vi "Create Core.vi"(6 "Custom Config Data":u8[](array[numeric]) format="%.0x", 7 "Direction":T2, 8 "error in (no error)":errorcluster, 9 "Disconnect Behavior":T1, 10 "Name":string, 11 "CIFChannels in":refnum<class "CIFChannels.lvclass">) -> (0 "error out":errorcluster, 3 "CIFChannels out":refnum<class "CIFChannels.lvclass">)   [LabVIEW 2021, in "CIFChannels.lvclass"]
uses:
  CIFChannels.lvclass
  Typedef/Direction.ctl
  Typedef/Disconnect Behavior.ctl
  Typedef/Channel State.ctl
  CIFChannels.lvclass/CIFChannels.ctl
  Accessors/Write Channel Class.vi
  Accessors/Write Channel State.vi
  Accessors/Write Direction.vi
  Accessors/Write Disconnect Behavior.vi
  Accessors/Write Name.vi
  Accessors/Write Custom Config Data.vi
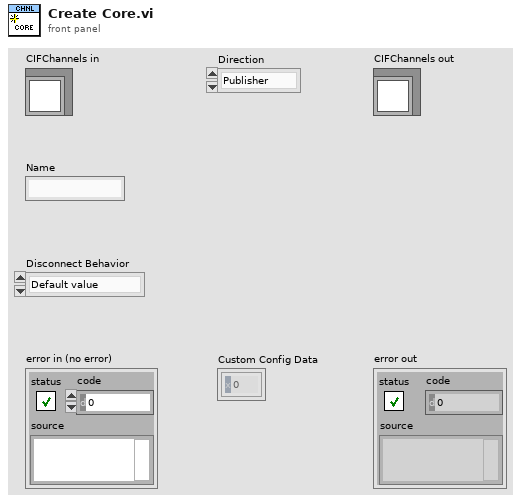
[diagram p1: front panel]
types:
  T1 = typedef "CIFChannels.lvclass/Disconnect Behavior.ctl" = enum16{"Default value", "Last value", "Error with default"}
  T2 = typedef "CIFChannels.lvclass/Direction.ctl" = enum16{"Publisher", "Subscriber"}
  T3 = typedef "CIFChannels.lvclass/Channel State.ctl" = enum16{"Creating", "Disconnected", "Connecting", "Connected", "Destroyed"}
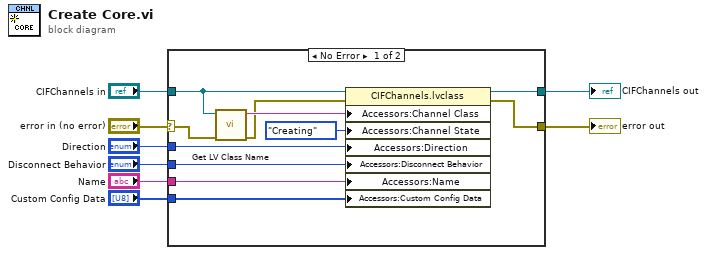
[diagram p0: block diagram]
diagram:
  n1 = case shown="No Error" "error in (no error)" {
    selector: "error in (no error)" -> [w11 w21]
    tunnel: [w18 w21] -> w7
    tunnel: [w19 w20] -> w5
    tunnel: "CIFChannels in" -> [w14 w20]
    tunnel: "Direction" -> [w17 _]
    tunnel: "Name" -> [w16 _]
    tunnel: "Disconnect Behavior" -> [w15 _]
    tunnel: "Custom Config Data" -> [w9 _]
    frame No Error {
      n2 = call <vilib>:"Get LV Class Name.vi"("error in (no error)"=w11, "object"=w14) -> ("error out"=w10:errorcluster, "class name"=w13:string)  [unwired: 8 in]
      n3 = property class="CIFChannels.lvclass"(reference=w14, error in=w10, "Accessors:Channel Class"=w13, "Accessors:Channel State"=Channel_State."Creating" ("Channel State"), "Accessors:Direction"=w17, "Accessors:Disconnect Behavior"=w15, "Accessors:Name"=w16, "Accessors:Custom Config Data"=w9) -> (reference out=w19:refnum<class "CIFChannels.lvclass">, error out=w18:errorcluster)
    }
    frame Error {
    }
  }
  "error out" <- w7
  "CIFChannels out" <- w5
